vi "log analysis_gps.vi"() -> ()   [LabVIEW 2018] (continued)
-1.000000000,38.289817810,-13.171142578,0.0,1.127054453,1.347936869,\"631T\",24,14,14,13,04,00,30,33*e902d0de\n\tsystem status\tnormal 0 28.300000 0 0\trobot status\t0.577126\t0.962583\t9.886100\t-0.042824\t-0.050098\t51.710182\t0.000000\t0.000000\n\t\n15:05:22.6\tlog_raw\tgps_raw\t\tsystem status\tnormal 0 28.400000 0 0\trobot status\t0.577700\t0.962351\t9.885900\t-0.041425\t-0.047478\t52.082989\t0.000000\t0.000000\n\t\n15:05:23.1\tlog_raw\tgps_raw\t#DUALANTENNAHEADINGA,USB3,0,46.5,FINESTEERING,2107,281141.100,02000000,d426,15824;SOL_COMPUTED,NARROW_INT,-1.000000000,38.544525146,-13.209045410,0.0,1.072585940,1.337732077,\"631T\",26,14,14,13,04,00,30,33*35811fe1\n\tsystem status\tnormal 0 28.400000 0 0\trobot status\t0.578980\t0.962091\t9.885800\t-0.040580\t-0.045830\t51.455475\t0.000000\t-0.001000\n\t\n15:05:23.6\tlog_raw\tgps_raw\t#DUALANTENNAHEADINGA,USB3,0,46.5,FINESTEERING,2107,281141.600,02000000,d426,15824;SOL_COMPUTED,NARROW_INT,-1.000000000,38.541603088,-13.618377686,0.0,1.070071220,1.342820048,\"631T\",26,14,14,13,04,00,20,33*482247c3\n\tsystem status\tnormal 0 28.400000 0 0\trobot status\t0.578613\t0.961856\t9.885900\t-0.040620\t-0.047974\t51.458397\t0.000000\t-0.001000\n\t\n15:05:24.1\tlog_raw\tgps_raw\t#DUALANTENNAHEADINGA,USB3,0,46.5,FINESTEERING,2107,281142.100,02000000,d426,15824;SOL_COMPUTED,NARROW_INT,-1.000000000,38.406040192,-13.289154053,0.0,1.036954045,1.309285402,\"631T\",27,14,14,13,04,00,30,33*cc93fd80\n\tsystem status\tnormal 0 28.300000 0 0\trobot status\t0.578395\t0.961497\t9.886100\t-0.040755\t-0.050298\t51.593960\t0.000000\t-0.001000\n\t\n15:05:24.6\tlog_raw\tgps_raw\t#DUALANTENNAHEADINGA,USB3,0,47.5,FINESTEERING,2107,281142.600,02000000,d426,15824;SOL_COMPUTED,NARROW_INT,-1.000000000,37.895870209,-13.180084229,0.0,0.624604940,0.826632023,\"631T\",28,18,18,13,04,00,30,33*963f3726\n\tsystem status\tnormal 0 28.300000 0 0\trobot status\t0.578368\t0.961329\t9.885800\t-0.039868\t-0.051662\t52.104130\t0.000000\t0.000000\n\t\n15:05:25.1\tlog_raw\tgps_raw\t#DUALANTENNAHEADINGA,USB3,0,42.0,FINESTEERING,2107,281143.100,02000000,d426,15824;SOL_COMPUTED,NARROW_INT,-1.000000000,38.331703186,-13.253448486,0.0,0.611471117,0.825593531,\"631T\",26,18,18,13,04,00,30,33*90346aac\n\tsystem status\tnormal 0 28.400000 0 0\trobot status\t0.578796\t0.961087\t9.885800\t-0.040433\t-0.051724\t51.668297\t0.000000\t0.000000\n\t\n15:05:25.6\tlog_raw\tgps_raw\t#DUALANTENNAHEADINGA,USB3,0,42.0,FINESTEERING,2107,281143.600,02000000,d426,15824;SOL_COMPUTED,NARROW_INT,-1.000000000,38.152809143,-13.672546387,0.0,0.610663354,0.814366698,\"631T\",26,18,18,13,04,00,30,33*9ca685c4\n\tsystem status\tnormal 0 28.400000 0 0\trobot status\t0.578630\t0.961052\t9.885700\t-0.039041\t-0.051583\t51.847191\t0.000000\t-0.001000\n\t\n15:05:26.1\tlog_raw\tgps_raw\t#DUALANTENNAHEADINGA,USB3,0,42.0,FINESTEERING,2107,281144.100,02000000,d426,15824;SOL_COMPUTED,NARROW_INT,-1.000000000,37.945987701,-13.233367920,0.0,0.669739842,0.855145931,\"631T\",26,18,18,13,04,00,30,33*123e83eb\n\tsystem status\tnormal 0 28.400000 0 0\trobot status\t0.578961\t0.960887\t9.885900\t-0.038586\t-0.052030\t52.054012\t0.000000\t0.000000\n\t\n15:05:26.6\tlog_raw\tgps_raw\t\tsystem status\tnormal 0 28.300000 0 0\trobot status\t0.578830\t0.960633\t9.885500\t-0.039530\t-0.054089\t52.211994\t0.000000\t-0.001000\n\t\n15:05:27.1\tlog_raw\tgps_raw\t#DUALANTENNAHEADINGA,USB3,0,45.0,FINESTEERING,2107,281145.100,02000000,d426,15824;SOL_COMPUTED,NARROW_INT,-1.000000000,37.653381348,-13.288238525,0.0,0.656995237,0.826921105,\"631T\",24,18,18,14,04,00,30,33*b472711d\n\tsystem status\tnormal 0 28.400000 0 0\trobot status\t0.579313\t0.960417\t9.885200\t-0.041146\t-0.054168\t52.346619\t0.000000\t0.000000\n\t\n15:05:27.6\tlog_raw\tgps_raw\t\tsystem status\tnormal 0 28.400000 0 0\trobot status\t0.578990\t0.960536\t9.885200\t-0.041842\t-0.055286\t52.157642\t0.000000\t0.000000\n\t\n15:05:28.1\tlog_raw\tgps_raw\t#DUALANTENNAHEADINGA,USB3,0,45.5,FINESTEERING,2107,281146.100,02000000,d426,15824;SOL_COMPUTED,NARROW_INT,-1.000000000,38.005626678,-12.970062256,0.0,0.727712393,0.990613818,\"631T\",25,15,15,14,04,00,20,33*86f1b1a8\n\tsystem status\tnormal 0 28.300000 0 0\trobot status\t0.579011\t0.960952\t9.885100\t-0.042144\t-0.056892\t51.994373\t0.000000\t0.000000\n\t\n15:05:28.6\tlog_raw\tgps_raw\t#DUALANTENNAHEADINGA,USB3,0,47.5,FINESTEERING,2107,281146.600,02000000,d426,15824;SOL_COMPUTED,NARROW_INT,-1.000000000,37.910751343,-12.991821289,0.0,0.759303749,1.121337056,\"631T\",25,18,18,14,04,00,30,33*44b276a0\n\tsystem status\tnormal 0 28.300000 0 0\trobot status\t0.578950\t0.960992\t9.885200\t-0.043335\t-0.054738\t52.089249\t0.000000\t-0.001000\n\t\n15:05:29.1\tlog_raw\tgps_raw\t\tsystem status\tnormal 0 28.300000 0 0\trobot status\t0.579357\t0.961191\t9.885600\t-0.042913\t-0.054015\t52.323448\t0.000000\t-0.001000\n\t\n15:05:29.6\tlog_raw\tgps_raw\t#DUALANTENNAHEADINGA,USB3,0,46.0,FINESTEERING,2107,281147.600,02000000,d426,15824;SOL_COMPUTED,NARROW_INT,-1.000000000,38.129638672,-13.341125488,0.0,0.886451721,1.098317146,\"631T\",25,15,15,14,04,00,20,33*a96005e6\n\tsystem status\tnormal 0 28.300000 0 0\trobot status\t0.578789\t0.961009\t9.885500\t-0.043336\t-0.053519\t51.870361\t0.000000\t0.000000\n\t\n15:05:30.1\tlog_raw\tgps_raw\t\tsystem status\tnormal 0 28.400000 0 0\trobot status\t0.578651\t0.960880\t9.885500\t-0.043246\t-0.051393\t52.201504\t0.000000\t0.000000\n\t\n15:05:30.6\tlog_raw\tgps_raw\t#DUALANTENNAHEADINGA,USB3,0,50.0,FINESTEERING,2107,281148.600,02000000,d426,15824;SOL_COMPUTED,NARROW_INT,-1.000000000,37.716373444,-13.426422119,0.0,0.669266760,0.970457733,\"631T\",24,17,17,14,04,00,30,33*2254214a\n\tsystem status\tnormal 0 28.400000 0 0\trobot status\t0.578369\t0.960736\t9.885400\t-0.042753\t-0.053282\t52.283627\t0.000000\t0.000000\n\t\n15:05:31.1\tlog_raw\tgps_raw\t\tsystem status\tnormal 0 28.400000 0 0\trobot status\t0.578794\t0.960694\t9.885500\t-0.044995\t-0.054801\t51.919659\t0.000000\t0.000000\n\t\n15:05:31.6\tlog_raw\tgps_raw\t#DUALANTENNAHEADINGA,USB3,0,47.0,FINESTEERING,2107,281149.600,02000000,d426,15824;SOL_COMPUTED,NARROW_INT,-1.000000000,37.979038239,-13.538208008,0.0,0.819728494,1.148574114,\"631T\",24,15,15,14,04,00,20,33*9d6d5ac5\n\tsystem status\tnormal 0 28.300000 0 0\trobot status\t0.578621\t0.960415\t9.885000\t-0.047677\t-0.054191\t52.020962\t0.000000\t-0.001000\n\t\n15:05:32.1\tlog_raw\tgps_raw\t\tsystem status\tnormal 0 28.300000 0 0\trobot status\t0.578706\t0.960495\t9.884900\t-0.047890\t-0.054397\t52.427273\t0.000000\t0.000000\n\t\n15:05:32.6\tlog_raw\tgps_raw\t#DUALANTENNAHEADINGA,USB3,0,49.5,FINESTEERING,2107,281150.600,02000000,d426,15824;SOL_COMPUTED,NARROW_INT,-1.000000000,37.228172302,-12.271484375,0.0,1.409551144,2.324419737,\"631T\",24,15,15,14,04,00,30,33*f37d2c86\n\tsystem status\tnormal 0 28.400000 0 0\trobot status\t0.578319\t0.960795\t9.884800\t-0.048539\t-0.053544\t52.771828\t0.000000\t0.000000\n\t\n15:05:33.1\tlog_raw\tgps_raw\t\tsystem status\tnormal 0 28.300000 0 0\trobot status\t0.578343\t0.961271\t9.885100\t-0.049245\t-0.053087\t52.220749\t0.000000\t0.000000\n\t\n15:05:33.6\tlog_raw\tgps_raw\t#DUALANTENNAHEADINGA,USB3,0,48.0,FINESTEERING,2107,281151.600,02000000,d426,15824;SOL_COMPUTED,NARROW_INT,-1.000000000,37.756275177,-12.401153564,0.0,0.810727656,2.464538813,\"631T\",25,15,15,14,04,00,30,33*0dea2661\n\tsystem status\tnormal 2 28.300000 0 0\trobot status\t0.580834\t0.965304\t9.885000\t-0.045800\t0.019332\t52.243725\t0.141000\t-0.038000\n\t\n15:05:34.1\tlog_raw\tgps_raw\t\tsystem status\tnormal 2 28.100000 0 0\trobot status\t0.703961\t1.130089\t9.886800\t-0.071833\t-0.085704\t51.125637\t0.516000\t-0.030000\n\t\n15:05:34.6\tlog_raw\tgps_raw\t#DUALANTENNAHEADINGA,USB3,0,45.0,FINESTEERING,2107,281152.600,02000000,d426,15824;SOL_COMPUTED,NARROW_INT,-1.000000000,41.067569733,-11.024108887,0.0,0.915120959,2.368236542,\"631T\",26,15,15,14,04,00,30,33*371e9095\n\tsystem status\tnormal 2 28.000000 0 0\trobot status\t0.851042\t1.314298\t9.891200\t0.074217\t-0.011053\t48.932430\t0.592000\t0.059000\n\t\n15:05:35.1\tlog_raw\tgps_raw\t\tsystem status\tnormal 2 27.900000 0 0\trobot status\t1.006625\t1.497370\t9.895400\t-0.225063\t0.106522\t46.853214\t0.645000\t0.177000\n\t\n15:05:35.6\tlog_raw\tgps_raw\t#DUALANTENNAHEADINGA,USB3,0,42.5,FINESTEERING,2107,281153.600,02000000,d426,15824;SOL_COMPUTED,NARROW_INT,-1.000000000,44.944766998,-11.911407471,0.0,1.110763311,1.443000793,\"631T\",25,14,14,12,04,00,20,33*620cb6bb\n\tsystem status\tnormal 2 27.900000 0 0\trobot status\t1.167677\t1.669002\t9.899300\t-0.305874\t0.198158\t45.055233\t0.449000\t-0.129000\n\t\n15:05:36.1\tlog_raw\tgps_raw\t#INSPVAXA,USB3,0,48.5,FINESTEERING,2107,281154.150,02000000,471d,15824;INS_ALIGNMENT_COMPLETE,INS_RTKFIXED,37.37014685396,126.72085037251,9.9046,22.3000,0.3217,0.3511,0.0243,-0.463440880,0.137300711,45.295089591,0.2336,0.1897,0.2924,0.0807,0.0781,0.0570,0.3153,0.3249,5.2966,0f000001,0*a5f38fa6\n\tsystem status\tnormal 2 28.000000 0 0\trobot status\t1.352363\t1.848720\t9.904600\t-0.463441\t0.137301\t42.629436\t0.442000\t-0.109000\n\t\n15:05:36.6\tlog_raw\tgps_raw\t#DUALANTENNAHEADINGA,USB3,0,48.5,FINESTEERING,2107,281154.600,02000000,d426,15824;SOL_COMPUTED,NARROW_INT,-1.000000000,49.660758972,-12.749389648,0.0,1.718050480,2.565145969,\"631T\",24,14,14,13,04,00,20,33*703fcd7f\n\tsystem status\tnormal 2 28.100000 0 0\trobot status\t1.508864\t1.989631\t9.908800\t-0.840754\t0.161600\t40.339241\t0.596000\t0.126000\n\t\n15:05:37.1\tlog_raw\tgps_raw\t#DUALANTENNAHEADINGA,USB3,0,46.5,FINESTEERING,2107,281155.100,02000000,d426,15824;SOL_COMPUTED,NARROW_INT,-1.000000000,50.095378876,-11.601318359,0.0,1.553679466,2.287994385,\"631T\",25,14,14,13,04,00,20,33*2e58f55a\n\tsystem status\tnormal 2 28.200000 0 0\trobot status\t1.685286\t2.137715\t9.914200\t-1.005580\t0.400573\t39.904621\t0.517000\t0.049000\n\t\n15:05:37.6\tlog_raw\tgps_raw\t\tsystem status\tnormal 2 28.300000 0 0\trobot status\t1.865443\t2.278902\t9.920400\t-0.937919\t0.362082\t38.911549\t0.470000\t-0.006000\n\t\n15:05:38.1\tlog_raw\tgps_raw\t#DUALANTENNAHEADINGA,USB3,0,46.5,FINESTEERING,2107,281156.100,02000000,d426,15824;SOL_COMPUTED,NARROW_INT,-1.000000000,50.991882324,-12.433105469,0.0,1.323938012,1.928015709,\"631T\",26,14,14,13,04,00,20,33*2250749f\n\tsystem status\tnormal 2 28.300000 0 0\trobot status\t2.040085\t2.410349\t9.926500\t-1.022467\t0.527268\t39.008118\t0.503000\t0.029000\n\t\n15:05:38.6\tlog_raw\tgps_raw\t#INSPVAXA,USB3,0,46.5,FINESTEERING,2107,281156.650,02000000,471d,15824;INS_ALIGNMENT_COMPLETE,INS_RTKFIXED,37.37015321622,126.72086040240,9.9343,22.3000,0.2996,0.4106,0.0140,-0.907814846,0.271069692,48.602781943,0.3009,0.2366,0.3431,0.1001,0.0915,0.0666,0.3160,0.3250,5.1102,0f000001,0*6f8cf050\n\tsystem status\tnormal 2 28.200000 0 0\trobot status\t2.240794\t2.554833\t9.934300\t-0.907815\t0.271070\t38.706905\t0.505000\t0.072000\n\t\n15:05:39.1\tlog_raw\tgps_raw\t#DUALANTENNAHEADINGA,USB3,0,44.5,FINESTEERING,2107,281157.100,02000000,d426,15824;SOL_COMPUTED,NARROW_INT,-1.000000000,50.954082489,-12.863372803,0.0,1.341279626,2.005761862,\"631T\",27,13,13,12,04,00,20,23*4fef6e2f\n\tsystem status\tnormal 2 28.300000 0 0\trobot status\t2.424831\t2.684836\t9.940800\t-0.614374\t0.109776\t39.045918\t0.474000\t0.067000\n\t\n15:05:39.6\tlog_raw\tgps_raw\t#DUALANTENNAHEADINGA,USB3,0,44.5,FINESTEERING,2107,281157.600,02000000,d426,15824;SOL_COMPUTED,NARROW_INT,-1.000000000,49.061492920,-13.071655273,0.0,1.635934353,2.562850237,\"631T\",26,11,11,10,04,00,20,03*548ab7b6\n\tsystem status\tnormal 2 28.000000 0 0\trobot status\t2.607588\t2.817131\t9.948000\t-0.729661\t0.223887\t40.938507\t0.414000\t0.211000\n\t\n15:05:40.1\tlog_raw\tgps_raw\t\tsystem status\tnormal 2 27.800000 0 0\trobot status\t2.787209\t2.952458\t9.955000\t-0.844215\t0.222466\t41.512199\t0.459000\t0.175000\n\t\n15:05:40.6\tlog_raw\tgps_raw\t#DUALANTENNAHEADINGA,USB3,0,45.5,FINESTEERING,2107,281158.600,02000000,d426,15824;SOL_COMPUTED,NARROW_INT,-1.000000000,45.442005157,-12.811401367,0.0,1.565847278,2.605268478,\"631T\",24,12,12,10,04,00,20,13*21c051c8\n\tsystem status\tnormal 2 27.700000 0 0\trobot status\t2.959785\t3.100779\t9.959600\t-0.949517\t-0.028380\t44.557995\t0.323000\t0.338000\n\t\n15:05:41.1\tlog_raw\tgps_raw\t#INSPVAXA,USB3,0,47.5,FINESTEERING,2107,281159.150,02000000,471d,15824;INS_ALIGNMENT_COMPLETE,INS_RTKFIXED,37.37015965988,126.72087054525,9.9670,22.3000,0.2751,0.2872,0.0208,-1.082759198,-0.090267714,39.552212675,0.3844,0.2766,0.4291,0.1130,0.0949,0.0735,0.3102,0.3164,4.9774,0f000001,0*4e2615f8\n\tsystem status\tnormal 2 27.700000 0 0\trobot status\t3.139231\t3.269980\t9.967000\t-1.082759\t-0.090268\t47.743134\t0.543000\t0.033000\n\t\n15:05:41.6\tlog_raw\tgps_raw\t\tsystem status\tnormal 2 27.700000 0 0\trobot status\t3.280830\t3.421960\t9.969400\t-1.052759\t-0.025260\t49.924076\t0.425000\t0.202000\n\t\n15:05:42.1\tlog_raw\tgps_raw\t#INSPVAXA,USB3,0,48.5,FINESTEERING,2107,281160.150,02000000,471d,15824;INS_ALIGNMENT_COMPLETE,INS_RTKFIXED,37.37016278311,126.72087401207,9.9722,22.3000,0.2922,0.2409,0.0084,-1.005101347,-0.168881236,34.455059248,0.3975,0.2811,0.4532,0.1112,0.0916,0.0745,0.3072,0.3124,4.9724,0f000001,0*0fce1499\n\tsystem status\tnormal 2 27.600000 0 0\trobot status\t3.446317\t3.616610\t9.972200\t-1.005101\t-0.168881\t52.567581\t0.485000\t0.083000\n\t\n15:05:42.6\tlog_raw\tgps_raw\t\tsystem status\tnormal 2 27.800000 0 0\trobot status\t3.569755\t3.784800\t9.976100\t-1.056865\t-0.255710\t55.497025\t0.467000\t0.093000\n\t\n15:05:43.1\tlog_raw\tgps_raw\t#DUALANTENNAHEADINGA,USB3,0,45.5,FINESTEERING,2107,281161.100,02000000,d426,15824;SOL_COMPUTED,NARROW_INT,-1.000000000,33.636985779,-10.703186035,0.0,1.305269480,1.988658309,\"631T\",23,10,10,9,04,00,20,03*63ae0eda\n\tsystem status\tnormal 2 27.800000 0 0\trobot status\t3.702715\t3.980108\t9.978200\t-1.012305\t-0.056747\t56.363014\t0.512000\t0.024000\n\t\n15:05:43.6\tlog_raw\tgps_raw\t#INSPVAXA,USB3,0,45.5,FINESTEERING,2107,281161.650,02000000,471d,15824;INS_ALIGNMENT_COMPLETE,INS_RTKFIXED,37.37016814009,126.72087850693,9.9782,22.3000,0.3668,0.2357,0.0033,-0.975313100,0.031183497,28.845006681,0.4039,0.2829,0.4738,0.1090,0.0894,0.0751,0.3046,0.3093,4.9734,0f000001,0*677f146d\n\tsystem status\tnormal 2 28.000000 0 0\trobot status\t3.844464\t4.211152\t9.978200\t-0.975313\t0.031183\t58.345957\t0.414000\t0.156000\n\t\n15:05:44.1\tlog_raw\tgps_raw\t\tsystem status\tnormal 2 28.000000 0 0\trobot status\t3.957509\t4.405304\t9.977800\t-0.939867\t-0.275378\t59.625040\t0.395000\t0.145000\n\t\n15:05:44.6\tlog_raw\tgps_raw\t#INSPVAXA,USB3,0,45.5,FINESTEERING,2107,281162.650,02000000,471d,15824;INS_ALIGNMENT_COMPLETE,INS_RTKFIXED,37.37017209764,126.72088131202,9.9740,22.3000,0.4165,0.2408,-0.0073,-0.889315400,-0.600255191,27.070811684,0.4059,0.2823,0.4897,0.1081,0.0892,0.0754,0.3028,0.3076,4.9743,0f000001,0*eec7da17\n\tsystem status\tnormal 2 28.100000 0 0\trobot status\t4.092934\t4.650379\t9.974000\t-0.889315\t-0.600255\t60.289593\t0.469000\t0.059000\n\t\n15:05:45.1\tlog_raw\tgps_raw\t\tsystem status\tnormal 2 28.200000 0 0\trobot status\t4.202474\t4.855213\t9.969900\t-0.753040\t-0.545938\t60.898582\t0.461000\t0.053000\n\t\n15:05:45.6\tlog_raw\tgps_raw\t#INSPVAXA,USB3,0,46.0,FINESTEERING,2107,281163.650,02000000,471d,15824;INS_ALIGNMENT_COMPLETE,INS_RTKFIXED,37.37017621040,126.72088401507,9.9622,22.3000,0.4228,0.2263,0.0028,-0.718735423,-0.648072833,26.654533136,0.4059,0.2813,0.5021,0.1087,0.0916,0.0754,0.3019,0.3070,4.9728,0f000001,0*7a23e206\n\tsystem status\tnormal 2 28.200000 0 0\trobot status\t4.332366\t5.106832\t9.962200\t-0.718735\t-0.648073\t60.667027\t0.471000\t0.022000\n\t\n15:05:46.1\tlog_raw\tgps_raw\t\tsystem status\tnormal 2 28.300000 0 0\trobot status\t4.438510\t5.311988\t9.955300\t-0.542305\t-0.526720\t60.004147\t0.498000\t-0.016000\n\t\n15:05:46.6\tlog_raw\tgps_raw\t#INSPVAXA,USB3,0,42.0,FINESTEERING,2107,281164.650,02000000,471d,15824;INS_ALIGNMENT_COMPLETE,INS_RTKFIXED,37.37018029891,126.72088666630,9.9494,22.3000,0.4427,0.2507,-0.0102,-0.527206458,-0.899456708,26.896972993,0.4048,0.2808,0.5108,0.1119,0.0963,0.0768,0.3015,0.3067,4.9703,0f000001,0*f7f5cf84\n\tsystem status\tnormal 2 28.300000 0 0\trobot status\t4.567208\t5.560593\t9.949400\t-0.527206\t-0.899457\t60.695930\t0.495000\t-0.037000\n\t\n15:05:47.1\tlog_raw\tgps_raw\t\tsystem status\tnormal 2 28.300000 0 0\trobot status\t4.677558\t5.773765\t9.943200\t-0.526821\t-0.977675\t60.043505\t0.492000\t-0.037000\n\t\n15:05:47.6\tlog_raw\tgps_raw\t#INSPVAXA,USB3,0,45.5,FINESTEERING,2107,281165.650,02000000,471d,15824;INS_ALIGNMENT_COMPLETE,INS_RTKFIXED,37.37018456715,126.72088948909,9.9368,22.3000,0.5066,0.2588,-0.0194,-0.465825854,-1.028181903,27.608896380,0.4043,0.2820,0.5169,0.1147,0.0992,0.0765,0.3012,0.3059,4.9676,0f000001,0*e22fcb74\n\tsystem status\tnormal 2 28.300000 0 0\trobot status\t4.817246\t6.034302\t9.936800\t-0.465826\t-1.028182\t60.516888\t0.505000\t-0.053000\n\t\n15:05:48.1\tlog_raw\tgps_raw\t\tsystem status\tnormal 2 28.300000 0 0\trobot status\t4.932791\t6.251339\t9.930600\t-0.468256\t-0.957865\t59.980766\t0.505000\t-0.035000\n\t\n15:05:48.6\tlog_raw\tgps_raw\t#INSPVAXA,USB3,0,45.5,FINESTEERING,2107,281166.650,02000000,471d,15824;INS_ALIGNMENT_COMPLETE,INS_RTKFIXED,37.37018872313,126.72089230644,9.9249,22.3000,0.5050,0.2695,-0.0048,-0.356872858,-0.951190565,28.973150163,0.4054,0.2841,0.5214,0.1194,0.1031,0.0797,0.3004,0.3038,4.9657,0f000001,0*e69e30b1\n\tsystem status\tnormal 2 28.100000 0 0\trobot status\t5.066802\t6.495552\t9.924900\t-0.356873\t-0.951191\t58.631643\t0.549000\t0.023000\n\t\n15:05:49.1\tlog_raw\tgps_raw\t#INSPVAXA,USB3,0,45.0,FINESTEERING,2107,281167.150,02000000,471d,15824;INS_ALIGNMENT_COMPLETE,INS_RTKFIXED,37.37019074562,126.72089375380,9.9189,22.3000,0.4684,0.2643,-0.0061,-0.477663869,-0.935450491,30.417591982,0.4082,0.2863,0.5249,0.1204,0.1022,0.0792,0.2990,0.3004,4.9651,0f000001,0*4f9f47ed\n\tsystem status\tnormal 2 28.000000 0 0\trobot status\t5.195007\t6.720017\t9.918900\t-0.477664\t-0.935450\t56.946583\t0.416000\t-0.172000\n\t\n15:05:49.6\tlog_raw\tgps_raw\t#INSPVAXA,USB3,0,45.0,FINESTEERING,2107,281167.650,02000000,471d,15824;INS_ALIGNMENT_COMPLETE,INS_RTKFIXED,37.37019269920,126.72089529645,9.9115,22.3000,0.4833,0.2919,-0.0020,-0.483216711,-1.218552457,32.463260828,0.4082,0.2863,0.5249,0.1204,0.1022,0.0792,0.2990,0.3004,4.9651,0f000001,0*7877b410\n\tsystem status\tnormal 2 28.000000 0 0\trobot status\t5.331652\t6.936834\t9.911500\t-0.483217\t-1.218552\t55.637012\t0.511000\t-0.043000\n\t\n15:05:50.1\tlog_raw\tgps_raw\t\tsystem status\tnormal 2 28.100000 0 0\trobot status\t5.457347\t7.121730\t9.907000\t-0.380181\t-0.970160\t53.132881\t0.554000\t0.028000\n\t\n15:05:50.6\tlog_raw\tgps_raw\t#INSPVAXA,USB3,0,45.5,FINESTEERING,2107,281168.650,02000000,471d,15824;INS_ALIGNMENT_COMPLETE,INS_RTKFIXED,37.37019633744,126.72089858847,9.9020,22.3000,0.4572,0.3119,0.0094,-0.439520835,-0.957492339,36.615351128,0.4109,0.2881,0.5277,0.1190,0.0994,0.0787,0.2969,0.2961,4.9653,0f000001,0*c67ea19b\n\tsystem status\tnormal 2 27.900000 0 0\trobot status\t5.623254\t7.340622\t9.902000\t-0.439521\t-0.957492\t51.308052\t0.681000\t0.185000\n\t\n15:05:51.1\tlog_raw\tgps_raw\t#INSPVAXA,USB3,0,41.5,FINESTEERING,2107,281169.150,02000000,471d,15824;INS_ALIGNMENT_COMPLETE,INS_RTKFIXED,37.37019803366,126.72090033617,9.8967,22.3000,0.4353,0.3466,-0.0124,-0.373798304,-0.691045943,38.520831977,0.4135,0.2910,0.5324,0.1162,0.0959,0.0784,0.2944,0.2920,4.9653,0f000001,0*85acc37f\n\tsystem status\tnormal 2 27.900000 0 0\trobot status\t5.778062\t7.528876\t9.896700\t-0.373798\t-0.691046\t48.554108\t0.450000\t-0.134000\n\t\n15:05:51.6\tlog_raw\tgps_raw\t#INSPVAXA,USB3,0,41.5,FINESTEERING,2107,281169.650,02000000,471d,15824;INS_ALIGNMENT_COMPLETE,INS_RTKFIXED,37.37019968370,126.72090219115,9.8910,22.3000,0.4092,0.3296,-0.0191,-0.608129529,-0.998598974,40.257706862,0.4135,0.2910,0.5324,0.1162,0.0959,0.0784,0.2944,0.2920,4.9653,0f000001,0*4e1130ac\n\tsystem status\tnormal 2 28.100000 0 0\trobot status\t5.942373\t7.712005\t9.891000\t-0.608130\t-0.998599\t47.946693\t0.451000\t-0.114000\n\t\n15:05:52.1\tlog_raw\tgps_raw\t#INSPVAXA,USB3,0,45.5,FINESTEERING,2107,281170.150,02000000,471d,15824;INS_ALIGNMENT_COMPLETE,INS_RTKFIXED,37.37020123427,126.72090408580,9.8830,22.3000,0.3824,0.3449,-0.0045,-0.472006885,-0.997512763,41.710684669,0.4139,0.2909,0.5351,0.1136,0.0932,0.0791,0.2920,0.2885,4.9641,0f000001,0*2dc0ad9b\n\tsystem status\tnormal 2 28.000000 0 0\trobot status\t6.110198\t7.884095\t9.883000\t-0.472007\t-0.997513\t46.620323\t0.571000\t0.093000\n\t\n15:05:52.6\tlog_raw\tgps_raw\t#INSPVAXA,USB3,0,45.5,FINESTEERING,2107,281170.650,02000000,471d,15824;INS_ALIGNMENT_COMPLETE,INS_RTKFIXED,37.37020269712,126.72090601410,9.8764,22.3000,0.3826,0.3439,-0.0555,-0.519783559,-1.040179137,42.895943819,0.4139,0.2909,0.5351,0.1136,0.0932,0.0791,0.2920,0.2885,4.9641,0f000001,0*7bedead2\n\tsystem status\tnormal 2 28.100000 0 0\trobot status\t6.281004\t8.046448\t9.876400\t-0.519784\t-1.040179\t44.978340\t0.411000\t-0.153000\n\t\n15:05:53.1\tlog_raw\tgps_raw\t#INSPVAXA,USB3,0,44.5,FINESTEERING,2107,281171.150,02000000,471d,15824;INS_ALIGNMENT_COMPLETE,INS_RTKFIXED,37.37020410008,126.72090794331,9.8693,22.3000,0.3861,0.3636,0.0003,-0.699793085,-1.013428627,43.781952509,0.4138,0.2914,0.5397,0.1111,0.0916,0.0789,0.2901,0.2864,4.9621,0f000001,0*75d8a529\n\tsystem status\tnormal 2 28.200000 0 0\trobot status\t6.451890\t8.202155\t9.869300\t-0.699793\t-1.013429\t44.127895\t0.402000\t-0.175000\n\t\n15:05:53.6\tlog_raw\tgps_raw\t#INSPVAXA,USB3,0,44.5,FINESTEERING,2107,281171.650,02000000,471d,15824;INS_ALIGNMENT_COMPLETE,INS_RTKFIXED,37.37020547941,126.72090993032,9.8591,22.3000,0.3712,0.3482,-0.0204,-0.626506310,-1.371933495,44.325085685,0.4138,0.2914,0.5397,0.1111,0.0916,0.0789,0.2901,0.2864,4.9621,0f000001,0*603a8c7d\n\tsystem status\tnormal 2 28.200000 0 0\trobot status\t6.627896\t8.355239\t9.859100\t-0.626506\t-1.371933\t43.276928\t0.411000\t-0.130000\n\t\n15:05:54.1\tlog_raw\tgps_raw\t#INSPVAXA,USB3,0,46.5,FINESTEERING,2107,281172.150,02000000,471d,15824;INS_ALIGNMENT_COMPLETE,INS_RTKFIXED,37.37020680132,126.72091185634,9.8504,22.3000,0.3423,0.3408,-0.0083,-0.892607382,-1.242115699,44.703288237,0.4137,0.2941,0.5475,0.1101,0.0921,0.0790,0.2889,0.2855,4.9595,0f000001,0*90544be8\n\tsystem status\tnormal 2 28.300000 0 0\trobot status\t6.798500\t8.501951\t9.850400\t-0.892607\t-1.242116\t43.027058\t0.482000\t-0.014000\n\t\n15:05:54.6\tlog_raw\tgps_raw\t#INSPVAXA,USB3,0,46.5,FINESTEERING,2107,281172.650,02000000,471d,15824;INS_ALIGNMENT_COMPLETE,INS_RTKFIXED,37.37020806274,126.72091379412,9.8428,22.3000,0.3393,0.3608,-0.0229,-0.508945363,-1.293654987,44.950159425,0.4137,0.2941,0.5475,0.1101,0.0921,0.0790,0.2889,0.2855,4.9595,0f000001,0*b56eb890\n\tsystem status\tnormal 2 28.300000 0 0\trobot status\t6.970145\t8.641949\t9.842800\t-0.508945\t-1.293655\t42.869167\t0.493000\t0.024000\n\t\n15:05:55.1\tlog_raw\tgps_raw\t#INSPVAXA,USB3,0,45.0,FINESTEERING,2107,281173.150,02000000,471d,15824;INS_ALIGNMENT_COMPLETE,INS_RTKFIXED,37.37020938618,126.72091581251,9.8332,22.3000,0.3324,0.3645,-0.0096,-0.521372580,-0.940346469,45.114108155,0.4131,0.2953,0.5536,0.1104,0.0943,0.0789,0.2883,0.2853,4.9566,0f000001,0*896df924\n\tsystem status\tnormal 2 28.300000 0 0\trobot status\t7.148931\t8.788830\t9.833200\t-0.521373\t-0.940346\t41.967030\t0.497000\t0.031000\n\t\n15:05:55.6\tlog_raw\tgps_raw\t#INSPVAXA,USB3,0,45.0,FINESTEERING,2107,281173.650,02000000,471d,15824;INS_ALIGNMENT_COMPLETE,INS_RTKFIXED,37.37021062105,126.72091771518,9.8279,22.3000,0.3141,0.3794,-0.0018,-0.763185421,-1.256731125,45.193767644,0.4131,0.2953,0.5536,0.1104,0.0943,0.0789,0.2883,0.2853,4.9566,0f000001,0*bce21ee6\n\tsystem status\tnormal 2 28.300000 0 0\trobot status\t7.317466\t8.925882\t9.827900\t-0.763185\t-1.256731\t42.092972\t0.497000\t0.014000\n\t\n15:05:56.1\tlog_raw\tgps_raw\t#INSPVAXA,USB3,0,42.5,FINESTEERING,2107,281174.150,02000000,471d,15824;INS_ALIGNMENT_COMPLETE,INS_RTKFIXED,37.37021196803,126.72091978453,9.8240,22.3000,0.3107,0.3301,0.0022,-0.763032701,-1.186677441,45.109324656,0.4135,0.2997,0.5622,0.1120,0.0966,0.0795,0.2881,0.2853,4.9521,0f000001,0*4885d5cd\n\tsystem status\tnormal 2 28.200000 0 0\trobot status\t7.500766\t9.075375\t9.824000\t-0.763033\t-1.186677\t42.113552\t0.512000\t0.015000\n\t\n15:05:56.6\tlog_raw\tgps_raw\t#INSPVAXA,USB3,0,42.5,FINESTEERING,2107,281174.650,02000000,471d,15824;INS_ALIGNMENT_COMPLETE,INS_RTKFIXED,37.37021324009,126.72092171742,9.8181,22.3000,0.3189,0.3639,-0.0177,-0.623768140,-1.260059850,44.385500285,0.4135,0.2997,0.5622,0.1120,0.0966,0.0795,0.2881,0.2853,4.9521,0f000001,0*5d7db614\n\tsystem status\tnormal 2 28.100000 0 0\trobot status\t7.671978\t9.216554\t9.818100\t-0.623768\t-1.260060\t42.845291\t0.378000\t0.202000\n\t\n15:05:57.1\tlog_raw\tgps_raw\t#INSPVAXA,USB3,0,46.0,FINESTEERING,2107,281175.150,02000000,471d,15824;INS_ALIGNMENT_COMPLETE,INS_RTKFIXED,37.37021454485,126.72092359431,9.8111,22.3000,0.2994,0.3285,-0.0007,-0.912779431,-1.090246712,43.056876175,0.4145,0.3032,0.5695,0.1139,0.0990,0.0803,0.2881,0.2850,4.9479,0f000001,0*1b591d65\n\tsystem status\tnormal 2 28.000000 0 0\trobot status\t7.838230\t9.361363\t9.811100\t-0.912779\t-1.090247\t43.990986\t0.394000\t0.233000\n\t\n15:05:57.6\tlog_raw\tgps_raw\t#INSPVAXA,USB3,0,46.0,FINESTEERING,2107,281175.650,02000000,471d,15824;INS_ALIGNMENT_COMPLETE,INS_RTKFIXED,37.37021589583,126.72092544139,9.8034,22.3000,0.3183,0.3129,-0.0016,-0.983600306,-1.421345156,41.411365334,0.4145,0.3032,0.5695,0.1139,0.0990,0.0803,0.2881,0.2850,4.9479,0f000001,0*27aaa3ef\n\tsystem status\tnormal 2 27.800000 0 0\trobot status\t8.001841\t9.511300\t9.803400\t-0.983600\t-1.421345\t45.491241\t0.549000\t-0.037000\n\t\n15:05:58.1\tlog_raw\tgps_raw\t#INSPVAXA,USB3,0,44.5,FINESTEERING,2107,281176.150,02000000,471d,15824;INS_ALIGNMENT_COMPLETE,INS_RTKFIXED,37.37021731136,126.72092726471,9.7967,22.3000,0.3067,0.3205,0.0018,-0.778712195,-1.421988866,39.539976805,0.4163,0.3059,0.5758,0.1149,0.0990,0.0812,0.2880,0.2842,4.9430,0f000001,0*48a96dd4\n\tsystem status\tnormal 2 28.000000 0 0\trobot status\t8.163348\t9.668402\t9.796700\t-0.778712\t-1.421989\t47.542530\t0.600000\t-0.072000\n\t\n15:05:58.6\tlog_raw\tgps_raw\t#INSPVAXA,USB3,0,44.5,FINESTEERING,2107,281176.650,02000000,471d,15824;INS_ALIGNMENT_COMPLETE,INS_RTKFIXED,37.37021874043,126.72092900172,9.7912,22.3000,0.3343,0.3105,-0.0118,-0.475424413,-1.033048404,37.733219685,0.4163,0.3059,0.5758,0.1149,0.0990,0.0812,0.2880,0.2842,4.9430,0f000001,0*63ca753e\n\tsystem status\tnormal 2 27.800000 0 0\trobot status\t8.317210\t9.827007\t9.791200\t-0.475424\t-1.033048\t48.924171\t0.262000\t0.419000\n\t\n15:05:59.1\tlog_raw\tgps_raw\t#INSPVAXA,USB3,0,46.0,FINESTEERING,2107,281177.150,02000000,471d,15824;INS_ALIGNMENT_COMPLETE,INS_RTKFIXED,37.37022027462,126.72093069920,9.7837,22.3000,0.3340,0.3056,-0.0059,-0.436029262,-1.318996825,36.094424232,0.4169,0.3052,0.5779,0.1146,0.0975,0.0816,0.2876,0.2828,4.9395,0f000001,0*8ee0afa4\n\tsystem status\tnormal 2 27.900000 0 0\trobot status\t8.467570\t9.997278\t9.783700\t-0.436029\t-1.318997\t50.639969\t0.587000\t-0.089000\n\t\n15:05:59.6\tlog_raw\tgps_raw\t#INSPVAXA,USB3,0,46.0,FINESTEERING,2107,281177.650,02000000,471d,15824;INS_ALIGNMENT_COMPLETE,INS_RTKFIXED,37.37022187937,126.72093233106,9.7786,22.3000,0.3383,0.3047,-0.0171,-0.416097585,-1.463260618,34.652814665,0.4169,0.3052,0.5779,0.1146,0.0975,0.0816,0.2876,0.2828,4.9395,0f000001,0*8906ebb7\n\tsystem status\tnormal 2 27.900000 0 0\trobot status\t8.612117\t10.175380\t9.778600\t-0.416098\t-1.463261\t52.582966\t0.431000\t0.144000\n\t\n15:06:00.1\tlog_raw\tgps_raw\t#INSPVAXA,USB3,0,43.5,FINESTEERING,2107,281178.150,02000000,471d,15824;INS_ALIGNMENT_COMPLETE,INS_RTKFIXED,37.37022350567,126.72093390601,9.7761,22.3000,0.3475,0.2828,-0.0164,-0.206861779,-1.246508732,33.446442474,0.4170,0.3028,0.5771,0.1137,0.0954,0.0819,0.2871,0.2813,4.9371,0f000001,0*562de2ee\n\tsystem status\tnormal 2 28.000000 0 0\trobot status\t8.751624\t10.355875\t9.776100\t-0.206862\t-1.246509\t53.900414\t0.496000\t0.041000\n\t\n15:06:00.6\tlog_raw\tgps_raw\t#INSPVAXA,USB3,0,43.5,FINESTEERING,2107,281178.650,02000000,471d,15824;INS_ALIGNMENT_COMPLETE,INS_RTKFIXED,37.37022519841,126.72093545972,9.7722,22.3000,0.3782,0.2868,-0.0191,-0.115839581,-1.073328137,32.590544637,0.4170,0.3028,0.5771,0.1137,0.0954,0.0819,0.2871,0.2813,4.9371,0f000001,0*73e5bb44\n\tsystem status\tnormal 2 28.100000 0 0\trobot status\t8.889249\t10.543742\t9.772200\t-0.115840\t-1.073328\t55.152020\t0.380000\t0.202000\n\t\n15:06:01.1\tlog_raw\tgps_raw\t#INSPVAXA,USB3,0,45.5,FINESTEERING,2107,281179.150,02000000,471d,15824;INS_ALIGNMENT_COMPLETE,INS_RTKFIXED,37.37022690987,126.72093697041,9.7680,22.3000,0.3622,0.2816,-0.0102,-0.207143991,-1.081874423,31.923591302,0.4160,0.2990,0.5741,0.1127,0.0939,0.0821,0.2866,0.2801,4.9362,0f000001,0*5c093e83\n\tsystem status\tnormal 2 28.100000 0 0\trobot status\t9.023063\t10.733688\t9.768000\t-0.207144\t-1.081874\t56.187019\t0.514000\t-0.020000\n\t\n15:06:01.6\tlog_raw\tgps_raw\t\tsystem status\tnormal 2 28.200000 0 0\trobot status\t9.161078\t10.932886\t9.763600\t-0.183128\t-1.227801\t56.129593\t0.642000\t-0.232000\n\t\n15:06:02.1\tlog_raw\tgps_raw\t#INSPVAXA,USB3,0,46.5,FINESTEERING,2107,281180.150,02008000,471d,15824;INS_ALIGNMENT_COMPLETE,INS_RTKFIXED,37.37023052669,126.72094007704,9.7564,22.3000,0.3610,0.2647,-0.0164,-0.513272391,-1.387154465,31.645867613,0.4155,0.2970,0.5730,0.1122,0.0935,0.0824,0.2863,0.2794,4.9359,0f000001,0*15d21dba\n\tsystem status\tnormal 2 28.300000 0 0\trobot status\t9.298243\t11.135099\t9.756400\t-0.513272\t-1.387154\t55.868034\t0.417000\t0.099000\n\t\n15:06:02.6\tlog_raw\tgps_raw\t#INSPVAXA,USB3,0,46.5,FINESTEERING,2107,281180.650,02008000,471d,15824;INS_ALIGNMENT_COMPLETE,INS_RTKFIXED,37.37023232250,126.72094161397,9.7484,22.3000,0.3885,0.2867,-0.0133,-0.410366705,-1.302704695,31.784927225,0.4155,0.2970,0.5730,0.1122,0.0935,0.0824,0.2863,0.2794,4.9359,0f000001,0*ecf83c2b\n\tsystem status\tnormal 2 28.300000 0 0\trobot status\t9.434382\t11.334406\t9.748400\t-0.410367\t-1.302705\t55.561245\t0.489000\t-0.006000\n\t\n15:06:03.1\tlog_raw\tgps_raw\t\tsystem status\tnormal 2 28.300000 0 0\trobot status\t9.571666\t11.533105\t9.740100\t-0.248954\t-1.461554\t54.766083\t0.485000\t-0.014000\n\t\n15:06:03.6\tlog_raw\tgps_raw\t#INSPVAXA,USB3,0,45.5,FINESTEERING,2107,281181.650,02008000,471d,15824;INS_ALIGNMENT_COMPLETE,INS_RTKFIXED,37.37023594976,126.72094471309,9.7312,22.3000,0.3923,0.2955,-0.0276,-0.429360160,-1.491752481,32.266896907,0.4140,0.2923,0.5675,0.1120,0.0932,0.0824,0.2861,0.2791,4.9367,0f000001,0*7730f092\n\tsystem status\tnormal 2 28.200000 0 0\trobot status\t9.708897\t11.736976\t9.731200\t-0.429360\t-1.491752\t54.639420\t0.494000\t-0.017000\n\t\n15:06:04.1\tlog_raw\tgps_raw\t\tsystem status\tnormal 2 28.200000 0 0\trobot status\t9.852150\t11.946030\t9.721600\t-0.359284\t-1.489124\t53.176060\t0.492000\t-0.017000\n\t\n15:06:04.6\tlog_raw\tgps_raw\t\tsystem status\tnormal 2 28.300000 0 0\trobot status\t9.993812\t12.156401\t9.716900\t-0.385078\t-1.348537\t54.688202\t0.493000\t-0.016000\n\t\n15:06:05.1\tlog_raw\tgps_raw\t#INSPVAXA,USB3,0,48.0,FINESTEERING,2107,281183.150,02008000,471d,15824;INS_ALIGNMENT_COMPLETE,INS_RTKFIXED,37.37024155075,126.72094950500,9.7123,22.3000,0.4055,0.2881,-0.0237,-0.200855406,-1.072709947,32.894593043,0.4104,0.2866,0.5571,0.1124,0.0939,0.0825,0.2862,0.2789,4.9396,0f000001,0*f844a638\n\tsystem status\tnormal 2 28.300000 0 0\trobot status\t10.133357\t12.358599\t9.712300\t-0.200855\t-1.072710\t54.295944\t0.499000\t-0.016000\n\t\n15:06:05.6\tlog_raw\tgps_raw\t\tsystem status\tnormal 2 28.300000 0 0\trobot status\t10.275319\t12.563251\t9.706900\t-0.577973\t-1.358056\t54.151482\t0.492000\t-0.028000\n\t\n15:06:06.1\tlog_raw\tgps_raw\t\tsystem status\tnormal 2 28.300000 0 0\trobot status\t10.420408\t12.767607\t9.702500\t-0.782350\t-1.294977\t54.118290\t0.494000\t-0.023000\n\t\n15:06:06.6\tlog_raw\tgps_raw\t#INSPVAXA,USB3,0,49.0,FINESTEERING,2107,281184.650,02008000,471d,15824;INS_ALIGNMENT_COMPLETE,INS_RTKFIXED,37.37024704588,126.72095439123,9.6966,22.3000,0.4339,0.3164,-0.0228,-0.832842396,-1.309145590,33.874103055,0.4098,0.2861,0.5540,0.1127,0.0942,0.0825,0.2862,0.2787,4.9412,0f000001,0*e6c1c908\n\tsystem status\tnormal 2 28.200000 0 0\trobot status\t10.566171\t12.968473\t9.696600\t-0.832842\t-1.309146\t53.540840\t0.505000\t-0.017000\n\t\n15:06:07.1\tlog_raw\tgps_raw\t\tsystem status\tnormal 2 28.300000 0 0\trobot status\t10.716919\t13.171333\t9.690300\t-0.789406\t-1.266538\t52.480869\t0.491000\t-0.011000\n\t\n15:06:07.6\tlog_raw\tgps_raw\t#INSPVAXA,USB3,0,44.5,FINESTEERING,2107,281185.650,02008000,471d,15824;INS_ALIGNMENT_COMPLETE,INS_RTKFIXED,37.37025062154,126.72095774565,9.6870,22.3000,0.4074,0.3266,-0.0025,-0.740348806,-1.419761740,34.752841376,0.4093,0.2853,0.5511,0.1123,0.0935,0.0817,0.2862,0.2784,4.9427,0f000001,0*da04eb84\n\tsystem status\tnormal 2 28.200000 0 0\trobot status\t10.863300\t13.365316\t9.687000\t-0.740349\t-1.419762\t51.453266\t0.506000\t-0.004000\n\t\n15:06:08.1\tlog_raw\tgps_raw\t\tsystem status\tnormal 2 28.300000 0 0\trobot status\t11.013966\t13.565453\t9.682200\t-1.088516\t-1.512449\t51.606689\t0.414000\t-0.106000\n\t\n15:06:08.6\tlog_raw\tgps_raw\t#INSPVAXA,USB3,0,46.0,FINESTEERING,2107,281186.650,02008000,471d,15824;INS_ALIGNMENT_COMPLETE,INS_RTKFIXED,37.37025416351,126.72096115786,9.6746,22.3000,0.3904,0.3327,-0.0338,-0.811943292,-1.291408071,35.723298207,0.4097,0.2868,0.5516,0.1126,0.0940,0.0823,0.2861,0.2778,4.9442,0f000001,0*aa987070\n\tsystem status\tnormal 2 28.200000 0 0\trobot status\t11.165548\t13.758420\t9.674600\t-0.811943\t-1.291408\t51.956127\t0.432000\t-0.116000\n\t\n15:06:09.1\tlog_raw\tgps_raw\t#INSPVAXA,USB3,0,42.0,FINESTEERING,2107,281187.150,02008000,471d,15824;INS_ALIGNMENT_COMPLETE,INS_RTKFIXED,37.37025583855,126.72096282892,9.6678,22.3000,0.4091,0.3516,-0.0259,-0.728228198,-1.245007299,36.027390494,0.4101,0.2875,0.5523,0.1126,0.0937,0.0826,0.2859,0.2773,4.9452,0f000001,0*776840fb\n\tsystem status\tnormal 2 28.300000 0 0\trobot status\t11.313568\t13.944323\t9.667800\t-0.728228\t-1.245007\t51.266438\t0.503000\t-0.008000\n\t\n15:06:09.6\tlog_raw\tgps_raw\t\tsystem status\tnormal 2 28.300000 0 0\trobot status\t11.463819\t14.130512\t9.663900\t-0.580791\t-1.011354\t51.095703\t0.491000\t-0.010000\n\t\n15:06:10.1\tlog_raw\tgps_raw\t#INSPVAXA,USB3,0,42.5,FINESTEERING,2107,281188.150,02000000,471d,15824;INS_ALIGNMENT_COMPLETE,INS_RTKFIXED,37.37025917986,126.72096621248,9.6609,22.3000,0.4052,0.3240,-0.0181,-0.745275066,-1.101586398,36.822015380,0.4109,0.2894,0.5546,0.1124,0.0934,0.0826,0.2858,0.2767,4.9465,0f000001,0*772ad5b2\n\tsystem status\tnormal 2 28.300000 0 0\trobot status\t11.613278\t14.315157\t9.660900\t-0.745275\t-1.101586\t51.216633\t0.495000\t-0.009000\n\t\n15:06:10.6\tlog_raw\tgps_raw\t\tsystem status\tnormal 2 28.300000 0 0\trobot status\t11.759026\t14.496605\t9.658900\t-0.990013\t-1.083592\t49.617485\t0.487000\t0.001000\n\t\n15:06:11.1\tlog_raw\tgps_raw\t#INSPVAXA,USB3,0,46.5,FINESTEERING,2107,281189.150,02000000,471d,15824;INS_ALIGNMENT_COMPLETE,INS_RTKFIXED,37.37026246505,126.72096957686,9.6575,22.3000,0.3818,0.3519,-0.0175,-0.837192728,-1.183881143,37.353641508,0.4111,0.2898,0.5556,0.1117,0.0925,0.0819,0.2856,0.2763,4.9479,0f000001,0*4984aef6\n\tsystem status\tnormal 2 28.300000 0 0\trobot status\t11.911289\t14.679762\t9.657500\t-0.837193\t-1.183881\t50.032913\t0.499000\t0.001000\n\t\n15:06:11.6\tlog_raw\tgps_raw\t\tsystem status\tnormal 2 28.300000 0 0\trobot status\t12.062375\t14.856372\t9.656100\t-0.598234\t-1.076823\t50.462673\t0.495000\t0.023000\n\t\n15:06:12.1\tlog_raw\tgps_raw\t#INSPVAXA,USB3,0,47.5,FINESTEERING,2107,281190.150,02000000,471d,15824;INS_ALIGNMENT_COMPLETE,INS_RTKFIXED,37.37026560808,126.72097291937,9.6539,22.3000,0.3854,0.3239,-0.0258,-0.774119778,-1.083116234,37.881716828,0.4108,0.2891,0.5553,0.1117,0.0926,0.0822,0.2854,0.2760,4.9491,0f000001,0*9066855d\n\tsystem status\tnormal 2 28.300000 0 0\trobot status\t12.207363\t15.028589\t9.653900\t-0.774120\t-1.083116\t49.671852\t0.490000\t0.013000\n\t\n15:06:12.6\tlog_raw\tgps_raw\t\tsystem status\tnormal 2 28.200000 0 0\trobot status\t12.365626\t15.217127\t9.648400\t-0.670855\t-1.220019\t49.869308\t0.496000\t0.012000\n\t\n15:06:13.1\tlog_raw\tgps_raw\t#INSPVAXA,USB3,0,46.5,FINESTEERING,2107,281191.150,02000000,471d,15824;INS_ALIGNMENT_COMPLETE,INS_RTKFIXED,37.37026891266,126.72097643520,9.6441,22.3000,0.4009,0.3345,-0.0087,-0.567088365,-1.086579521,38.077503099,0.4100,0.2882,0.5540,0.1113,0.0920,0.0813,0.2854,0.2758,4.9504,0f000001,0*a8ef7184\n\tsystem status\tnormal 2 28.300000 0 0\trobot status\t12.518790\t15.395346\t9.644100\t-0.567088\t-1.086580\t49.336937\t0.506000\t0.018000\n\t\n15:06:13.6\tlog_raw\tgps_raw\t\tsystem status\tnormal 2 28.200000 0 0\trobot status\t12.668491\t15.565771\t9.639700\t-0.472166\t-0.814924\t50.367130\t0.487000\t0.028000\n\t\n15:06:14.1\tlog_raw\tgps_raw\t\tsystem status\tnormal 2 28.200000 0 0\trobot status\t12.820296\t15.742116\t9.635800\t-0.471136\t-1.040344\t50.941689\t0.613000\t-0.176000\n\t\n15:06:14.6\tlog_raw\tgps_raw\t\tsystem status\tnormal 2 28.100000 0 0\trobot status\t12.967058\t15.918267\t9.635000\t-0.344302\t-0.820499\t51.399658\t0.485000\t0.057000\n\t\n15:06:15.1\tlog_raw\tgps_raw\t\tsystem status\tnormal 2 28.100000 0 0\trobot status\t13.110101\t16.097778\t9.633200\t-0.471213\t-1.066021\t51.720249\t0.434000\t0.100000\n\t\n15:06:15.6\tlog_raw\tgps_raw\t#INSPVAXA,USB3,0,44.5,FINESTEERING,2107,281193.650,02000000,471d,15824;INS_ALIGNMENT_COMPLETE,INS_RTKFIXED,37.37027685595,126.72098468760,9.6314,22.3000,0.3773,0.2845,-0.0187,-0.353904451,-0.860332510,34.629255191,0.4086,0.2861,0.5496,0.1111,0.0919,0.0805,0.2853,0.2756,4.9528,0f000001,0*0c511912\n\tsystem status\tnormal 2 28.000000 0 0\trobot status\t13.249774\t16.276928\t9.631400\t-0.353904\t-0.860333\t53.095947\t0.643000\t-0.218000\n\t\n15:06:16.1\tlog_raw\tgps_raw\t\tsystem status\tnormal 2 28.100000 0 0\trobot status\t13.387336\t16.462578\t9.629400\t-0.353561\t-1.177931\t53.450153\t0.397000\t0.170000\n\t\n15:06:16.6\tlog_raw\tgps_raw\t\tsystem status\tnormal 2 28.000000 0 0\trobot status\t13.523546\t16.652185\t9.627100\t-0.146678\t-1.203958\t54.566383\t0.508000\t0.030000\n\t\n15:06:17.1\tlog_raw\tgps_raw\t#INSPVAXA,USB3,0,45.0,FINESTEERING,2107,281195.150,02000000,471d,15824;INS_ALIGNMENT_COMPLETE,INS_RTKFIXED,37.37028195184,126.72098923738,9.6233,22.3000,0.3859,0.2758,0.0067,-0.277560926,-1.244099586,32.051440833,0.4079,0.2838,0.5437,0.1122,0.0928,0.0817,0.2853,0.2754,4.9558,0f000001,0*9827a4c3\n\tsystem status\tnormal 2 28.100000 0 0\trobot status\t13.652786\t16.842492\t9.623300\t-0.277561\t-1.244100\t55.884487\t0.441000\t0.099000\n\t\n15:06:17.6\tlog_raw\tgps_raw\t\tsystem status\tnormal 2 28.200000 0 0\trobot status\t13.781939\t17.036936\t9.618300\t-0.255448\t-1.246733\t55.940342\t0.466000\t0.059000\n\t\n15:06:18.1\tlog_raw\tgps_raw\t\tsystem status\tnormal 2 28.200000 0 0\trobot status\t13.909337\t17.231040\t9.612400\t0.000672\t-1.288653\t57.245113\t0.632000\t-0.210000\n\t\n15:06:18.6\tlog_raw\tgps_raw\t\tsystem status\tnormal 2 28.200000 0 0\trobot status\t14.036028\t17.431243\t9.609100\t-0.324754\t-1.474202\t57.401436\t0.696000\t-0.301000\n\t\n15:06:19.1\tlog_raw\tgps_raw\t\tsystem status\tnormal 2 28.200000 0 0\trobot status\t14.160799\t17.628274\t9.603800\t-0.385686\t-1.306239\t56.606216\t0.410000\t0.132000\n\t\n15:06:19.6\tlog_raw\tgps_raw\t\tsystem status\tnormal 2 28.200000 0 0\trobot status\t14.288276\t17.826743\t9.597400\t-0.052299\t-0.953857\t56.838486\t0.548000\t-0.100000\n\t\n15:06:20.1\tlog_raw\tgps_raw\t\tsystem status\tnormal 2 28.300000 0 0\trobot status\t14.416248\t18.032677\t9.591600\t-0.284518\t-1.109191\t56.558506\t0.480000\t0.004000\n\t\n15:06:20.6\tlog_raw\tgps_raw\t\tsystem status\tnormal 2 28.300000 0 0\trobot status\t14.541438\t18.234059\t9.585500\t-0.585127\t-1.023591\t56.100204\t0.502000\t-0.013000\n\t\n15:06:21.1\t
